vi "Connect_PS1-_GND.vi"(3 "error in":errorcluster) -> (10 "error out":errorcluster)   [LabVIEW 2015]
panel:
  # "ON means close relay\nOFF means open relay"
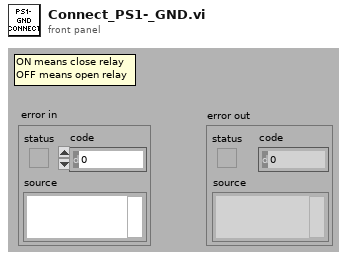
[diagram p1: front panel]
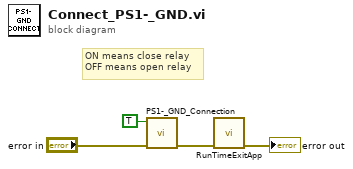
[diagram p0: block diagram]
diagram:
  # "ON means close relay\nOFF means open relay"
  n1 = call "PS1-_GND_Connection.vi"("On/Off"=TRUE, "error in"="error in") -> ("error out"=w2:errorcluster)  [unwired: 8 in]
  n2 = call "RunTimeExitApp.vi"("error in (no error)"=w2) -> ("error out"=→"error out":errorcluster)  [unwired: 10 in]
